vi "Test Missing VIs.vi"(8 "error in":errorcluster, 11 "My Computer":refnum<vi>) -> (0 "error out":errorcluster, 4 "Missing items":path[](array[path]), 5 "Pass":bool, 6 "Debug":path[](array[path]))   [LabVIEW 2020, in "Missing in Project Tests.lvlib"]
doc: "Tests to make sure all VIs and Ctls defined in the project are saved to disk."
uses:
  Missing in Project Tests.lvlib
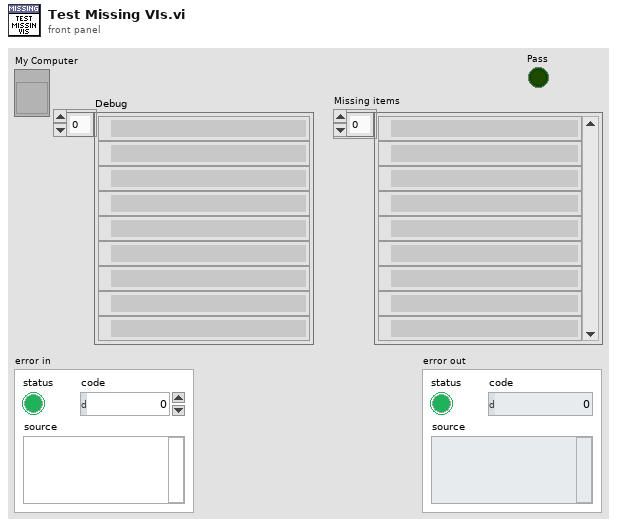
[diagram p1: front panel]
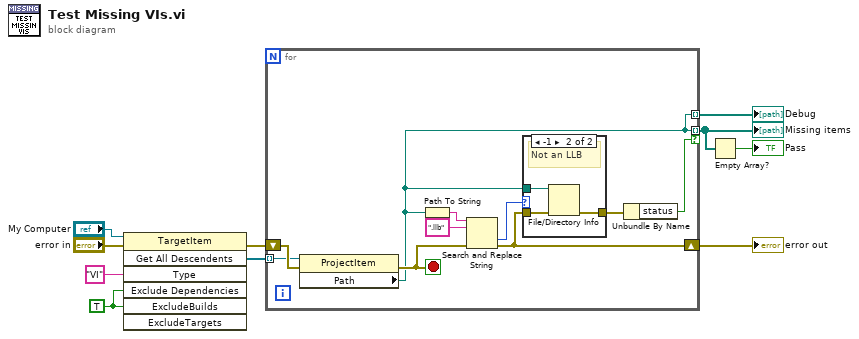
[diagram p0: block diagram]
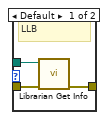
[diagram p2: hidden frame]
diagram:
  w3 = TRUE ("ExcludeBuilds")
  n1 = invoke on="Invoke Node" class="TargetItem" method="Get All Descendents"(reference="My Computer", error in="error in", "Type"="VI", "Exclude Dependencies"=w3, "ExcludeBuilds"=w3) -> (error out=w10:errorcluster, "All Descendents"=w6:refnum<vi>[])  [unwired: 2 in, 5 out]
  n2 = for {
    tunnel: w6 -> [w16] mode=indexing
    shift-right: [w17] -> w9
    shift-left: w10 -> [w19]
    tunnel: [w11] -> w5 mode=indexing if=w15
    tunnel: [w11] -> w1 mode=indexing
    stop <- w18 stop-if-true
    n3 = property on="Property Node" class="ProjectItem"(reference=w16, error in=w19) -> (error out=w18:errorcluster, "Path"=w11:path)  [unwired: 1 out]
    n4 = Path To String(path=w11) -> (string=w14:string)
    n5 = Search and Replace String(input string=w14, search string=".llb", error in=w18) -> (offset past replacement=w12:i32, error out=w17:errorcluster)  [unwired: 5 in, 2 out]
    n6 = case shown="-1" w12 {
      tunnel: w17 -> [w23 w26]
      tunnel: [w22 w25] -> w20
      tunnel: w11 -> [w21 w24]
      frame Default {
        # "LLB"
        n7 = call <vilib>:"Librarian Get Info.vi"("error in (no error)"=w23, "path"=w21) -> ("error out"=w22:errorcluster)  [unwired: 7 in, 2 out]
      }
      frame -1 {
        # "Not an LLB"
        n8 = File/Directory Info(path=w24, error in=w26) -> (error out=w25:errorcluster)  [unwired: 6 out]
      }
    }
    n9 = Unbundle By Name(w20) -> ("status"=w15:bool)
  }
  "Missing items" <- w5
  "error out" <- w9
  "Debug" <- w1
  n10 = Empty Array?(array=w5) -> (empty?=→"Pass":bool)
